vi "serial.vi"() -> ()   [LabVIEW 2014]
panel:
  out "波形チャート":dbl(graph)
  out "読み取りバッファ":string
  in  "停止":bool
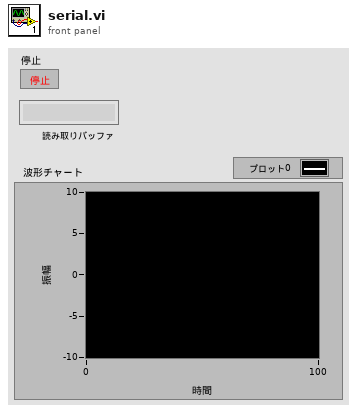
[diagram p1: front panel]
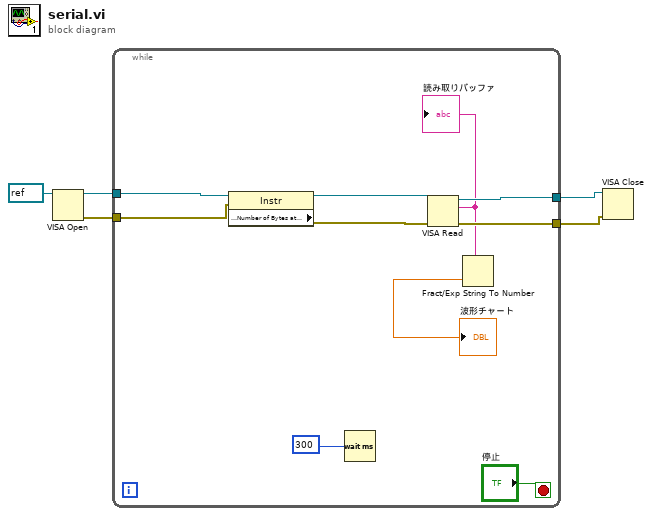
[diagram p0: block diagram]
diagram:
  n1 = VISA Open(VISA resource name=refnum<visa-resource-name> refnum ("VISAリソース名")) -> (VISA resource name=w5:refnum<visa-resource-name>, error out=w4:errorcluster)  [unwired: 4 in]
  n2 = while {
    tunnel: w5 -> [w13]
    tunnel: w4 -> [w12]
    tunnel: [w10] -> w3
    tunnel: [w8] -> w2
    stop <- "停止" stop-if-true
    n3 = property class="Instr" props=["Serial Settings:Number of Bytes at Serial Port"](reference=w13, error in=w12) -> (reference out=w11:refnum<visa-resource-name>, error out=w9:errorcluster)  [unwired: 1 out]
    n4 = Wait (ms)(milliseconds to wait=u32 300 ("ミリ秒待機時間")) -> ()  [unwired: 1 out]
    n5 = VISA Read(VISA resource name=w11, error in (no error)=w9) -> (VISA resource name out=w10:refnum<visa-resource-name>, read buffer=w7:string, error out=w8:errorcluster)  [unwired: 1 in, 1 out]
    "読み取りバッファ" <- w7
    n6 = Fract/Exp String To Number(string=w7) -> (number=→"波形チャート":dbl)  [unwired: 3 in, 1 out]
  }
  n7 = VISA Close(VISA resource name=w3, error in (no error)=w2) -> ()  [unwired: 1 out]
